vi "Configure Channel (OHM Normal).vi"(0 "VISA resource name":refnum<visa-resource-name>, 5 "Channel (0001)":string="0001", 7 "Enable Channel (True)":bool=TRUE, 9 "Type and Span":T1={"OHM Type (0 : 20ohm)"=0, "Enable Span (False)"=FALSE, "Lower Span (0.000)"=0.0, "Upper Span (20.000)"=20.0, "Bias (0)"=0.0} {"Bias (0)" format="%_6g"; "Upper Span (20.000)" min=-99999.0 max=99999.0 step=0.1 format="%.2f"; "Lower Span (0.000)" min=-99999.0 max=99999.0 step=0.1 format="%.2f"; "OHM Type (0 : 20ohm)" items=["20ohm", "200ohm", "2000ohm"]}, 11 "error in (no error)":errorcluster) -> (4 "VISA resource name out":refnum<visa-resource-name>, 6 "Channel":string, 15 "error out":errorcluster)   [LabVIEW 2020, in "Yokogawa GX Series.lvlib"]
doc: "Sets the input range as OHM (for 4 wire RTD).\n\nCommand: SRangeAI"
uses:
  <instrlib>/Yokogawa GX Series/Yokogawa GX Series.lvlib
  <instrlib>/Yokogawa GX Series/Private/OHM Range.vi
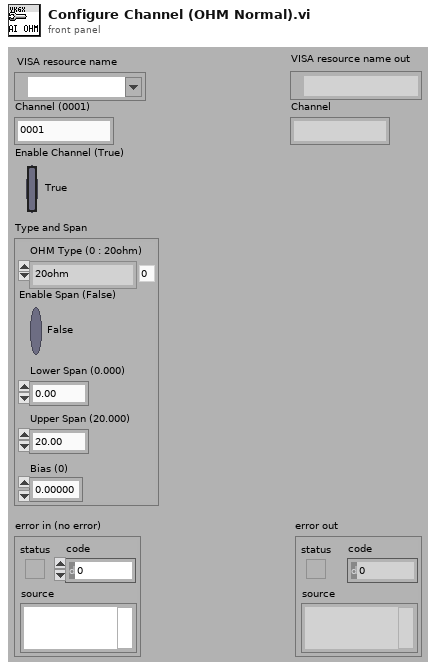
[diagram p1: front panel]
types:
  T1 = cluster{"OHM Type (0 : 20ohm)":i32, "Enable Span (False)":bool, "Lower Span (0.000)":dbl, "Upper Span (20.000)":dbl, "Bias (0)":dbl}
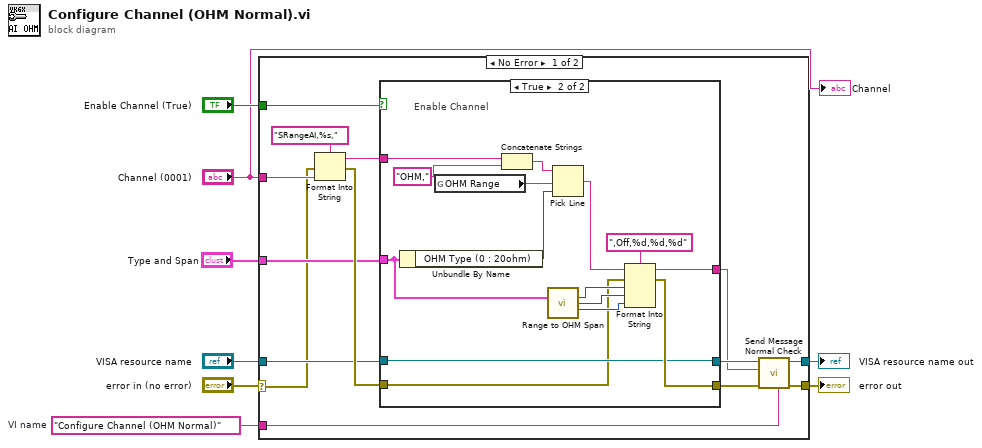
[diagram p0: block diagram]
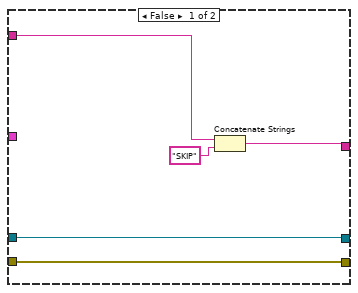
[diagram p2: hidden frame]
diagram:
  w3 = "Configure Channel (OHM Normal)"  # VI name
  n1 = case shown="No Error" "error in (no error)" {
    selector: "error in (no error)" -> [w9 w43]
    tunnel: "Enable Channel (True)" -> [w19 _]
    tunnel: "VISA resource name" -> [w18 w44]
    tunnel: "Type and Span" -> [w17 _]
    tunnel: [w13 w44] -> w5
    tunnel: [w12 w43] -> w4
    tunnel: w3 -> [w11 _]
    tunnel: "Channel (0001)" -> [w10 _]
    frame No Error {
      n2 = Format Into String(format string="SRangeAI,%s,", error in=w9, w10) -> (resulting string=w20:string, error out=w21:errorcluster)  [unwired: 1 in]
      n3 = case shown="True" w19 {
        tunnel: w21 -> [w26 w30]
        tunnel: w20 -> [w27 w41]
        tunnel: [w26 w40] -> w15
        tunnel: w18 -> [w25 w31]
        tunnel: [w25 w31] -> w16
        tunnel: w17 -> [_ w38]
        tunnel: [w23 w35] -> w14
        frame False {
          n4 = Concatenate Strings(w27, "SKIP") -> (w23:string)
        }
        frame True {
          # "Enable Channel"
          n5 = Unbundle By Name(w38) -> ("OHM Type (0 : 20ohm)"=w37:i32)
          n6 = global read "OHM Range.vi" "OHM Range"() -> (w28:string)
          n7 = Concatenate Strings(w41, "OHM,") -> (w39:string)
          n8 = call <instrlib>:"Range to OHM Span.vi"("Range And Span"=w38) -> ("Lower Span"=w34:i32, "Upper Span"=w33:i32, "Bias"=w32:i32)  [unwired: 12 in]
          n9 = Pick Line(string ("")=w39, multi-line string=w28, line index=w37) -> (output string=w36:string)
          n10 = Format Into String(format string=",Off,%d,%d,%d", initial string=w36, error in=w30, w34, w33, w32) -> (resulting string=w35:string, error out=w40:errorcluster)
        }
      }
      n11 = call <instrlib>:"Send Message Normal Check.vi"("Source (\"\")"=w11, "error in (no error)"=w15, "Send Message (\"\")"=w14, "VISA resource name"=w16) -> ("error out"=w12:errorcluster, "VISA resource name out"=w13:refnum<visa-resource-name>)  [unwired: 2 in, 4 out]
    }
    frame Error {
    }
  }
  "error out" <- w4
  "VISA resource name out" <- w5
  "Channel" <- "Channel (0001)"
